vi "Fpga-Get-Integer8.vi"(7 "lower":u16=2, 9 "Reset":bool, 10 "DataIn":u8, 11 "Index":u16) -> (2 "Valid":bool, 3 "U8":u8)   [LabVIEW 2016]
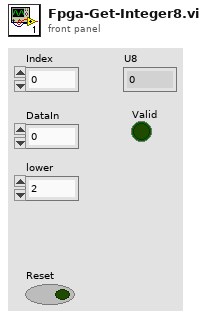
[diagram p1: front panel]
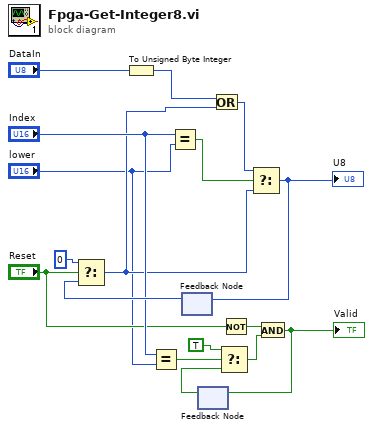
[diagram p0: block diagram]
diagram:
  n1 = To Unsigned Byte Integer(number="DataIn") -> (unsigned 8bit integer=w13:u8)
  n2 = Equal?(x="Index", y="lower") -> (x = y?=w10:bool)
  n3 = Equal?(x="Index", y="lower") -> (x = y?=w3:bool)
  n4 = feedback #1() -> (w16:u8)  [unwired: 1 in]
  n5 = Select(t=u8 0, s="Reset", f=w16) -> (s? t:f=w2:u8)
  n6 = feedback #2() -> (w8:bool)  [unwired: 1 in]
  n7 = Or(x=w13, y=w2) -> (x .or. y?=w12:u8)
  n8 = Select(t=TRUE, s=w10, f=w8) -> (s? t:f=w5:bool)
  n9 = Not(x="Reset") -> (.not. x?=w6:bool)
  n10 = Select(t=w12, s=w3, f=w2) -> (s? t:f=w15:u8)
  "U8" <- w15
  n11 = feedback-in #1(w15) -> ()
  n12 = And(x=w6, y=w5) -> (x .and. y?=w4:bool)
  "Valid" <- w4
  n13 = feedback-in #2(w4) -> ()
